vi "createMultiReaderBuilder.vi"(8 "error in (no error)":errorcluster) -> (0 "error out":errorcluster, 3 "IMultiReaderBuilder out":refnum<class "IMultiReaderBuilder.lvclass">)   [LabVIEW 2022 SP3, in "openDAQ.lvlib" / "IBaseObject.lvlib" / "IMultiReaderBuilder.lvlib" / "IMultiReaderBuilder.lvclass"]
uses:
  <instrlib>/openDAQ/Public/Classes/IMultiReaderBuilder/IMultiReaderBuilder.lvclass
  C:/Program Files (x86)/National Instruments/LabVIEW 2022/instr.lib/openDAQ/Public/Classes/IBaseObject/IBaseObject.lvclass
  <instrlib>/openDAQ/Public/Classes/IBaseObject/IBaseObject.lvclass/IBaseObject.ctl
  <instrlib>/openDAQ/Public/Classes/IBaseObject/Accessor/Read reference.vi
  <instrlib>/openDAQ/Public/Classes/IBaseObject/Accessor/Write reference.vi
  <instrlib>/openDAQ/Binaries/Windows/x86/copendaq32.dll
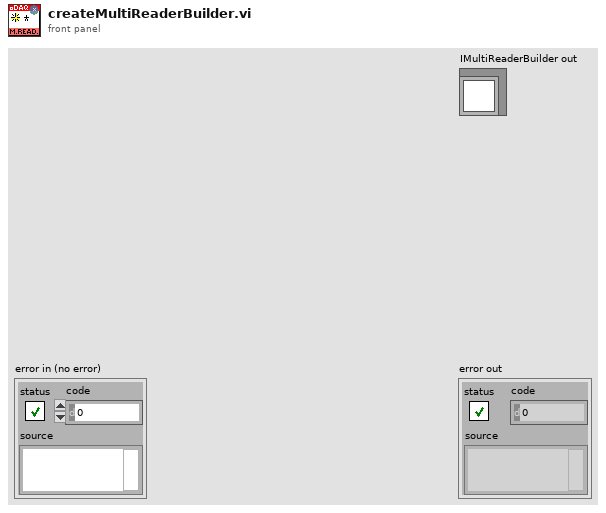
[diagram p1: front panel]
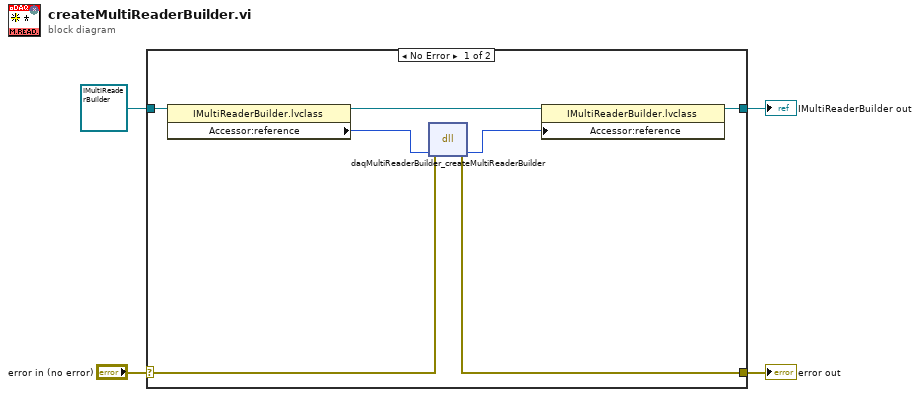
[diagram p0: block diagram]
diagram:
  n1 = case shown="No Error" "error in (no error)" {
    selector: "error in (no error)" -> [w10 w13]
    tunnel: [w9 w13] -> w3
    tunnel: [w7 w12] -> w1
    tunnel: refnum<class "IMultiReaderBuilder.lvclass"> refnum ("IMultiReaderBuilder in") -> [w11 w12]
    frame No Error {
      n2 = property class="IMultiReaderBuilder.lvclass"(reference=w11) -> (reference out=w8:refnum<class "IMultiReaderBuilder.lvclass">, "Accessor:reference"=w6:i64)  [unwired: 1 in, 1 out]
      n3 = dll-call lib="C:/Program Files (x86)/National Instruments/LabVIEW 2022/instr.lib/openDAQ/Binaries/Windows/x86/copendaq*.*" fn="daqMultiReaderBuilder_createMultiReaderBuilder"(error in=w10, "builder"=w6) -> (error out=w9:errorcluster, "builder"=w5:i64)  [unwired: 3 in, 1 out]
      n4 = property class="IMultiReaderBuilder.lvclass"(reference=w8, "Accessor:reference"=w5) -> (reference out=w7:refnum<class "IMultiReaderBuilder.lvclass">)  [unwired: 1 in, 1 out]
    }
    frame Error {
    }
  }
  "error out" <- w3
  "IMultiReaderBuilder out" <- w1
